vi "Default Configuration Parameters.vi"() -> (3 "Default Configuration":T1)   [LabVIEW 2020, in "RandomNumberLogger.lvlib" / "RandomNumberLogger.lvclass"]
doc: "<b>Default Configuration Parameters</b>\nThis VI allows you to define default parameter values for your plugin. These defaults will be loaded by the configuration utility when you add this plugin to a configuration."
uses:
  RandomNumberLogger.lvclass
  RandomNumberLogger.lvclass/RandomNumberLogger.ctl
  Configuration.ctl
panel:
  # "#via_ignore"
  # "** Updates must be made on block diagram **"
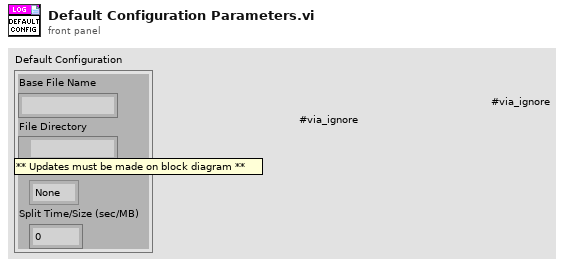
[diagram p1: front panel]
types:
  T1 = typedef "RandomNumberLogger.lvlib/RandomNumberLogger.lvclass/Configuration.ctl" = cluster{"Base File Name":string, "File Directory":path, "File Split":enum16{"None", "Time", "Size"}, "Split Time/Size (sec/MB)":dbl}
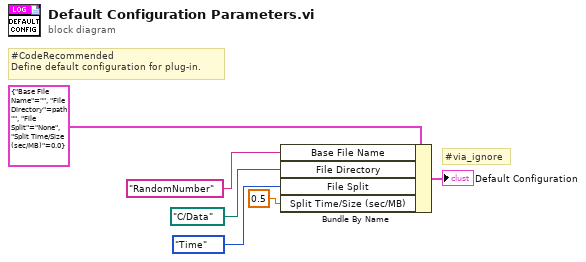
[diagram p0: block diagram]
diagram:
  # "#via_ignore"
  # "#CodeRecommended\nDefine default configuration for plug-in."
  n1 = Bundle By Name(cluster=T1 {"Base File Name"="", "File Directory"=path "", "File Split"=enum."None", "Split Time/Size (sec/MB)"=0.0} ("Default Configuration"), "Base File Name"="RandomNumber", "File Directory"=path "C:/Data", "File Split"=enum16{"None", "Time", "Size"}."Time", "Split Time/Size (sec/MB)"=0.5) -> (→"Default Configuration":T1)
